vi "Timer Action Engine.vi"(8 "error in (no error)":errorcluster, 11 "Action":T1) -> (0 "error out":errorcluster, 3 "Current time (ms)":u32)   [LabVIEW 2020]
doc: "FGV to monitor the time elapsed for the timed acquisition."
uses:
  controls/Timer AE states ---typedef.ctl
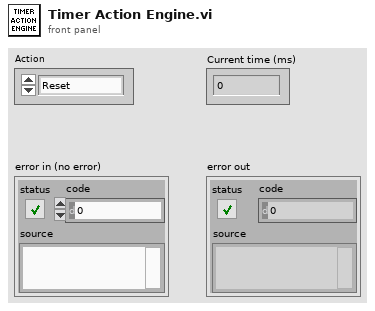
[diagram p1: front panel]
types:
  T1 = typedef "Timer AE states ---typedef.ctl" = enum16{"Reset", "Get", "Pause", "Continue"}
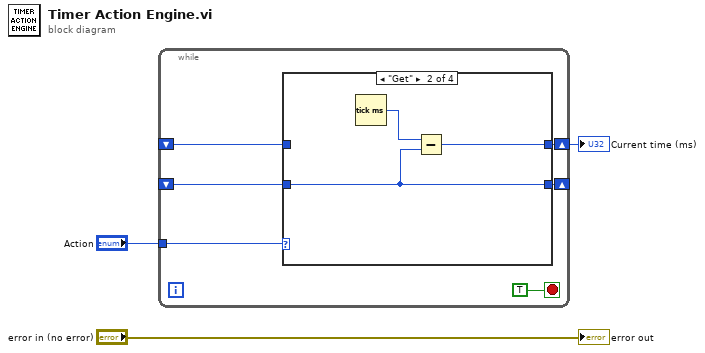
[diagram p0: block diagram]
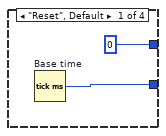
[diagram p2: hidden frame]
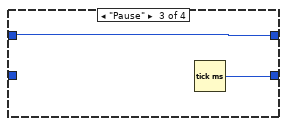
[diagram p3: hidden frame]
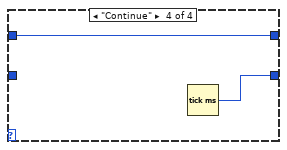
[diagram p4: hidden frame]
diagram:
  n1 = while {
    tunnel: "Action" -> [w8]
    shift-right: [w7] -> _
    shift-left: _ -> [w6]
    shift-right: [w5] -> w2
    shift-left: _ -> [w4]
    stop <- TRUE stop-if-true
    n2 = case shown="\"Get\"" w8 {
      tunnel: [w11 w13 w15 w17] -> w7
      tunnel: w6 -> [_ w13 _ _]
      tunnel: [u32 0 w12 w16 w18] -> w5
      tunnel: w4 -> [_ _ w16 w18]
      frame "Reset", Default {
        n3 = Tick Count (ms) "Base time"() -> (millisecond timer value=w11:u32)
      }
      frame "Get" {
        n4 = Tick Count (ms)() -> (millisecond timer value=w14:u32)
        n5 = Subtract(x=w14, y=w13) -> (x-y=w12:u32)
      }
      frame "Pause" {
        n6 = Tick Count (ms)() -> (millisecond timer value=w15:u32)
      }
      frame "Continue" {
        n7 = Tick Count (ms)() -> (millisecond timer value=w17:u32)
      }
    }
  }
  "Current time (ms)" <- w2
  "error out" <- "error in (no error)"
